vi "Write Channels_ Reference.vi"(8 "error in (no error)":errorcluster, 10 "Configuration.Channels: REF":T1 {"Roll-Off" min=1; "TC" min=0.0001 format="%#_3p"; "Phase" format="%.3g"; "Frequency" min=0.0001 max=10000.0 format="%.3g"}, 11 "Lockin.DAQ":refnum<class "Instrument.DAQ.lvclass">) -> (0 "error out":errorcluster, 3 "Lockin.DAQ out":refnum<class "Instrument.DAQ.lvclass">)   [LabVIEW 2019, in "Instrument.DAQ.lvclass"]
uses:
  Instrument.DAQ.lvclass
  Typedefs/REF-cluster.ctl
  Instrument UI.Lockin/Typedefs/REF Channel--Cluster.ctl
  Instrument.DAQ.lvclass/Instrument.DAQ.ctl
  Instrument UI.Lockin/Instrument UI.Lockin.lvclass
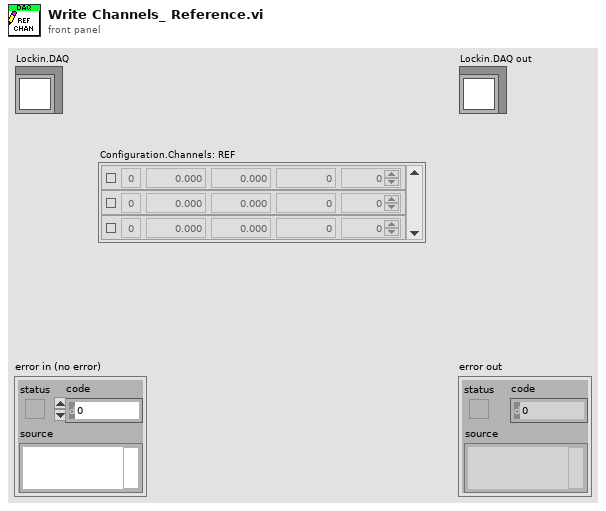
[diagram p1: front panel]
types:
  T1 = typedef "Instrument.DAQ.lvclass/REF-cluster.ctl" = T2[]
  T2 = typedef "Instrument UI.Lockin.lvclass/REF Channel--Cluster.ctl" = cluster{"Enable?":bool, "Channel":i32, "Frequency":dbl, "Phase":dbl, "TC":dbl, "Roll-Off":i32}
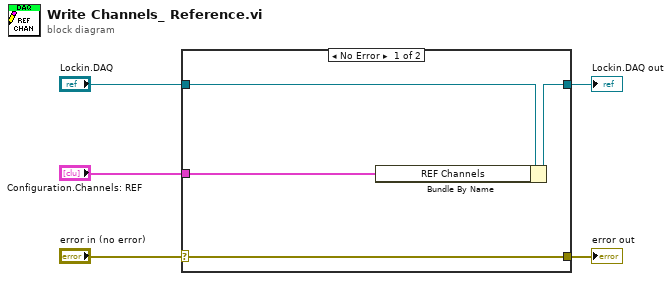
[diagram p0: block diagram]
diagram:
  n1 = case shown="No Error" "error in (no error)" {
    selector: "error in (no error)" -> [w9 w10]
    tunnel: [w9 w10] -> w4
    tunnel: [w6 w11] -> w2
    tunnel: "Lockin.DAQ" -> [w8 w11]
    tunnel: "Configuration.Channels: REF" -> [w7 _]
    frame No Error {
      n2 = Bundle By Name(cluster=w8, "REF Channels"=w7) -> (w6:refnum<class "Instrument.DAQ.lvclass">)
    }
    frame Error {
    }
  }
  "error out" <- w4
  "Lockin.DAQ out" <- w2
